vi "transmitterwazeer.vi"() -> ()   [LabVIEW 2020]
uses:
  <vilib>/Analysis/3filter.llb/Filter Passband Type.ctl
  <vilib>/Analysis/baseanly.llb/Mean (DBL).vi
  <vilib>/Utility/file.llb/Read Delimited Spreadsheet (DBL).vi
  <vilib>/Analysis/3filter.llb/Butterworth Filter (DBL).vi
  <instrlib>/niUSRP/niUSRP Write Tx Data (2D CDB).vi
  <vilib>/Utility/file.llb/Write Delimited Spreadsheet (DBL).vi
  <vilib>/Analysis/NI_AALBase.lvlib
  <vilib>/Analysis/NI_AAL_SigProc.lvlib
panel:
  in  "active antenna":string
  in  "gain":dbl format="%#_6f"
  in  "carrier frequency":dbl=100000.0 format="%#_6p"
  in  "IQ rate":dbl=100000.0 format="%#_6p"
  in  "device names":refnum<k15>
  in  "sampling freq: fs":dbl=1000.0 format="%0.2f"
  in  "low cutoff freq: fl":dbl(slide)=4.790874524714829 scale=0.0..50.0
  in  "Tab Control":T1(tab)
  out "Waveform Graph":dbl[](graph)
  out "Waveform Graph 2":dbl[](graph)
  out "Waveform Graph 3":dbl[](graph)
  out "Waveform Graph 4":dbl[](graph)
  out "Waveform Graph 5":dbl[](graph)
  out "Waveform Graph 6":dbl[](graph)
  out "Waveform Graph 7":dbl[](graph)
  out "Waveform Graph 8":dbl[](graph)
  out "Waveform Graph 9":dbl[][](graph)
  out "Waveform Graph 10":dbl[][](graph)
  out "Array":i32[](array[numeric])
  in  "stop":bool
  in  "file path (dialog if empty)":path
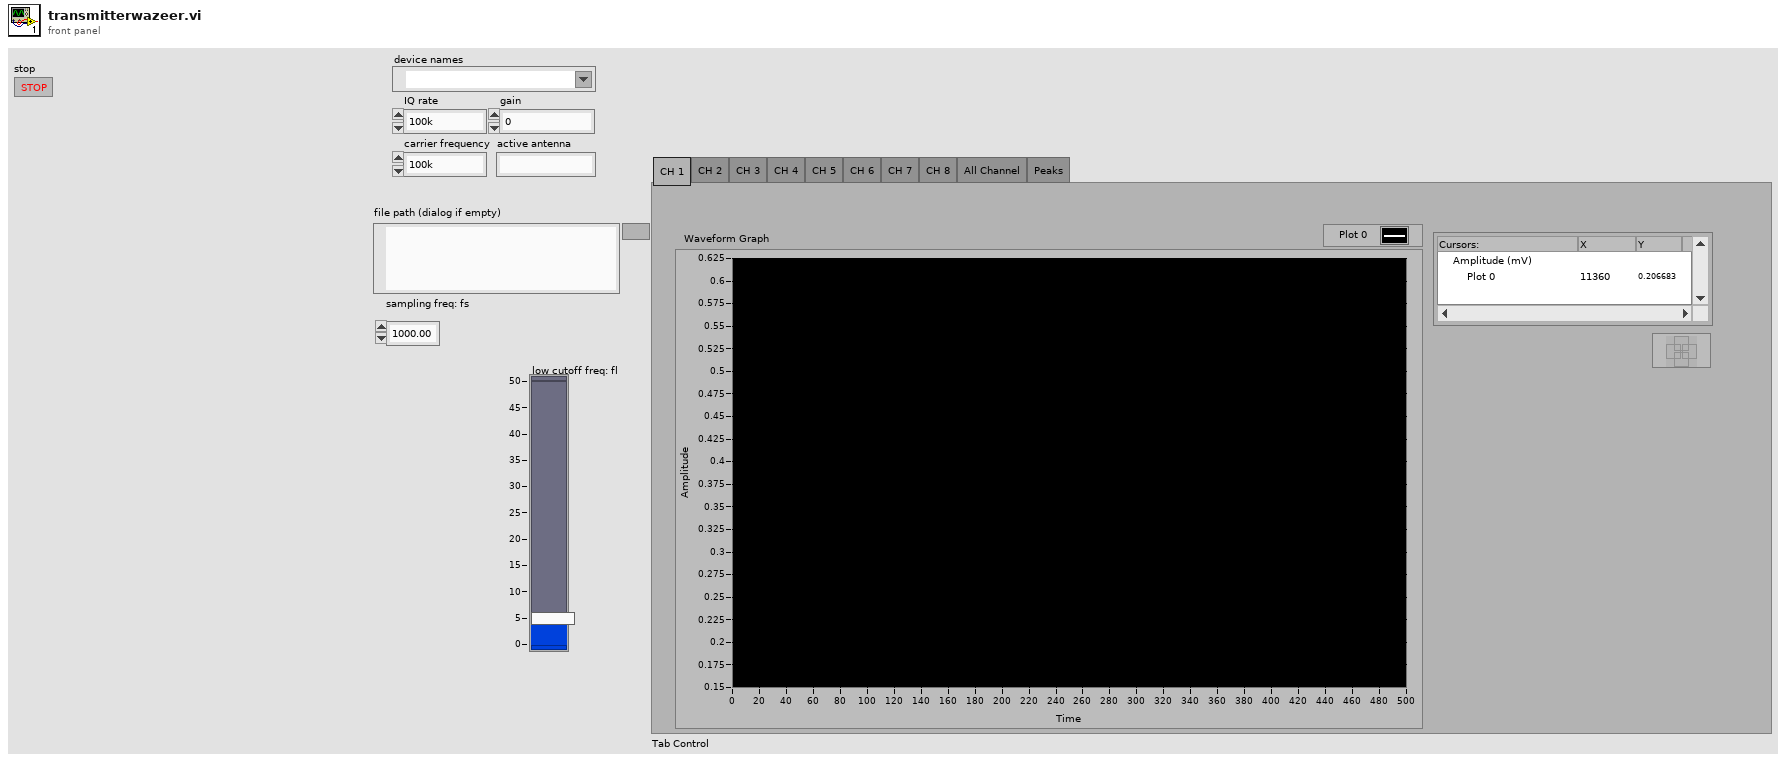
[diagram p1: front panel]
types:
  T1 = enum32{"CH 1", "CH 2", "CH 3", "CH 4", "CH 5", "CH 6", "CH 7", "CH 8", "All Channel", "Peaks"}
  T2 = typedef "NI_AALBase.lvlib/Filter Passband Type.ctl" = enum32{"Lowpass", "Highpass", "Bandpass", "Bandstop"}
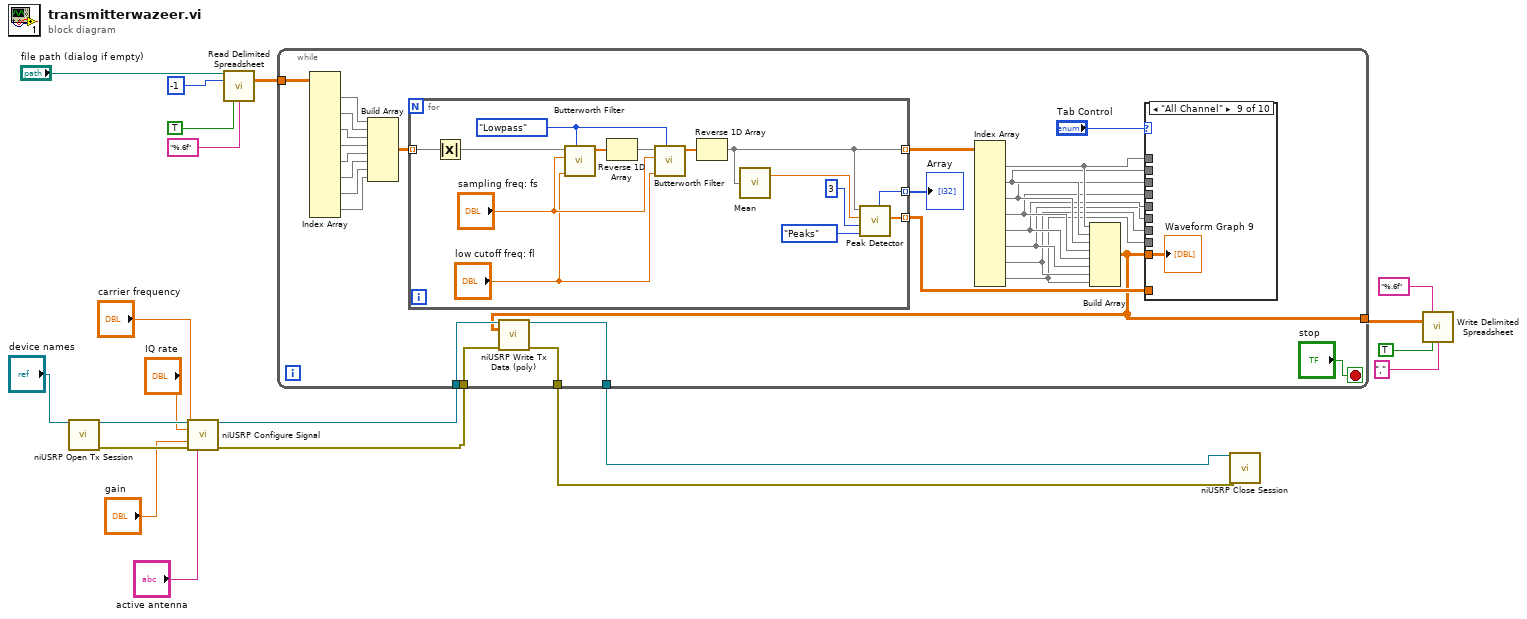
[diagram p0: block diagram]
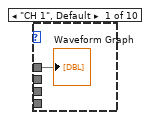
[diagram p2: hidden frame]
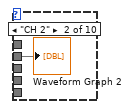
[diagram p3: hidden frame]
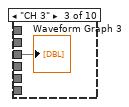
[diagram p4: hidden frame]
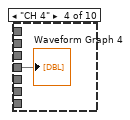
[diagram p5: hidden frame]
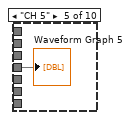
[diagram p6: hidden frame]
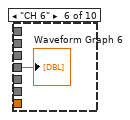
[diagram p7: hidden frame]
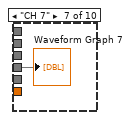
[diagram p8: hidden frame]
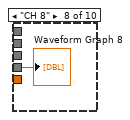
[diagram p9: hidden frame]
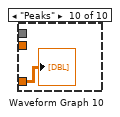
[diagram p10: hidden frame]
diagram:
  n1 = call <instrlib>:"niUSRP Open Tx Session.vi"("device names"="device names") -> ("session handle out"=w11:refnum<k15>, "error out"=w10:errorcluster)  [unwired: 13 in]
  n2 = call <instrlib>:"niUSRP Configure Signal.vi"("session handle"=w11, "IQ rate"="IQ rate", "carrier frequency"="carrier frequency", "gain"="gain", "error in (no error)"=w10, "active antenna"="active antenna") -> ("session handle out"=w9:refnum<k15>, "error out"=w8:errorcluster)  [unwired: 5 in, 3 out]
  n3 = call-poly <vilib>:"Read Delimited Spreadsheet.vi"("file path (dialog if empty)"="file path (dialog if empty)", "number of rows (all:-1)"=-1, "transpose? (F)"=TRUE, "delimiter (\\t)"="%.6f" ("delimiter (\\t)")) -> ("all rows"=w16:dbl[][])  [unwired: 6 in, 5 out]
  n4 = while {
    tunnel: w16 -> [w48]
    tunnel: [w21] -> w12
    tunnel: w9 -> [w25]
    tunnel: w8 -> [w24]
    tunnel: [w23] -> w7
    tunnel: [w22] -> w6
    stop <- "stop" stop-if-true
    n5 = Index Array "Index Array"(array=w48) -> (element #1=w47:dbl[], element #2=w46:dbl[], element #3=w45:dbl[], element #4=w44:dbl[], element #5=w43:dbl[], element #6=w42:dbl[], element #7=w41:dbl[], element #8=w40:dbl[])  [unwired: 16 in]
    n6 = Build Array "Build Array"(w47, w46, w45, w44, w43, w42, w41, w40) -> (w39:dbl[][])
    n7 = for {
      tunnel: w39 -> [w72] mode=indexing
      tunnel: [w61] -> w38 mode=indexing
      tunnel: [w60] -> w37 mode=indexing
      tunnel: [w59] -> w27 mode=indexing
      w67 = Filter_Passband_Type."Lowpass" ("filter type")
      n8 = Absolute Value(x=w72) -> (abs(x)=w68:dbl[])
      n9 = call-poly <vilib>:"Butterworth Filter.vi"("filter type"=w67, "low cutoff freq: fl"="low cutoff freq: fl", "sampling freq: fs"="sampling freq: fs", "X"=w68) -> ("Filtered X"=w71:dbl[])  [unwired: 4 in, 1 out]
      n10 = Reverse 1D Array(array=w71) -> (reversed array=w69:dbl[])
      n11 = call-poly <vilib>:"Butterworth Filter.vi"("filter type"=w67, "low cutoff freq: fl"="low cutoff freq: fl", "sampling freq: fs"="sampling freq: fs", "X"=w69) -> ("Filtered X"=w70:dbl[])  [unwired: 4 in, 1 out]
      n12 = Reverse 1D Array(array=w70) -> (reversed array=w61:dbl[])
      n13 = call-poly <vilib>:"Mean.vi"("X"=w61) -> ("mean"=w64:dbl)  [unwired: 1 out]
      n14 = call <vilib>:"Peak Detector.vi"("peaks/valleys"=enum32{"Peaks", "Valleys"}."Peaks", "width"=3, "threshold"=w64, "X"=w61) -> ("Amplitudes"=w59:dbl[], "# found"=w60:i32)  [unwired: 3 in, 3 out]
    }
    "Array" <- w37
    n15 = Index Array(array=w38) -> (element #1=w35:dbl[], element #2=w34:dbl[], element #3=w33:dbl[], element #4=w32:dbl[], element #5=w31:dbl[], element #6=w30:dbl[], element #7=w29:dbl[], element #8=w28:dbl[])  [unwired: 16 in]
    n16 = Build Array(w35, w34, w33, w32, w31, w30, w29, w28) -> (w21:dbl[][])
    n17 = call-poly <instrlib>:"niUSRP Write Tx Data (poly).vi"("session handle"=w25, "data"=w21, "error in (no error)"=w24) -> ("session handle out"=w22:refnum<k15>, "error out"=w23:errorcluster)  [unwired: 11 in]
    n18 = case shown="\"All Channel\"" "Tab Control" {
      tunnel: w35 -> [w49 _ _ _ _ _ _ _ _ _]
      tunnel: w34 -> [_ w50 _ _ _ _ _ _ _ _]
      tunnel: w33 -> [_ _ w51 _ _ _ _ _ _ _]
      tunnel: w32 -> [_ _ _ w52 _ _ _ _ _ _]
      tunnel: w31 -> [_ _ _ _ w53 _ _ _ _ _]
      tunnel: w30 -> [_ _ _ _ _ w54 _ _ _ _]
      tunnel: w29 -> [_ _ _ _ _ _ w55 _ _ _]
      tunnel: w28 -> [_ _ _ _ _ _ _ w56 _ _]
      tunnel: w21 -> [_ _ _ _ _ _ _ _ w57 _]
      tunnel: w27 -> [_ _ _ _ _ _ _ _ _ w58]
      frame "CH 1", Default {
        "Waveform Graph" <- w49
      }
      frame "CH 2" {
        "Waveform Graph 2" <- w50
      }
      frame "CH 3" {
        "Waveform Graph 3" <- w51
      }
      frame "CH 4" {
        "Waveform Graph 4" <- w52
      }
      frame "CH 5" {
        "Waveform Graph 5" <- w53
      }
      frame "CH 6" {
        "Waveform Graph 6" <- w54
      }
      frame "CH 7" {
        "Waveform Graph 7" <- w55
      }
      frame "CH 8" {
        "Waveform Graph 8" <- w56
      }
      frame "All Channel" {
        "Waveform Graph 9" <- w57
      }
      frame "Peaks" {
        "Waveform Graph 10" <- w58
      }
    }
  }
  n19 = call <instrlib>:"niUSRP Close Session.vi"("session handle"=w6, "error in (no error)"=w7) -> ()  [unwired: 13 in, 1 out]
  n20 = call-poly <vilib>:"Write Delimited Spreadsheet.vi"("format (%.3f)"="%.6f", "2D data"=w12, "transpose? (no:F)"=TRUE, "delimiter (\\t)"="," ("delimiter (\\t)")) -> ()  [unwired: 10 in, 2 out]
